vi "Word Wrap License File.vi"(8 "error in":errorcluster, 11 "txt file path":path) -> (0 "error out":errorcluster)   [LabVIEW 2011]
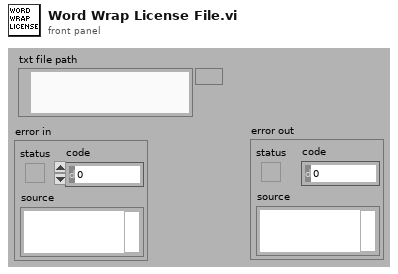
[diagram p1: front panel]
types:
  T1 = enum16{"User-specified Font", "Application Font", "System Font", "Dialog Font"}
  T2 = cluster{"Font Name:":string, "Size":i16, "Strikeout?":bool, "Italic?":bool, "Underline?":bool, "Outline?":bool, "Shadow?":bool, "Bold?":bool}
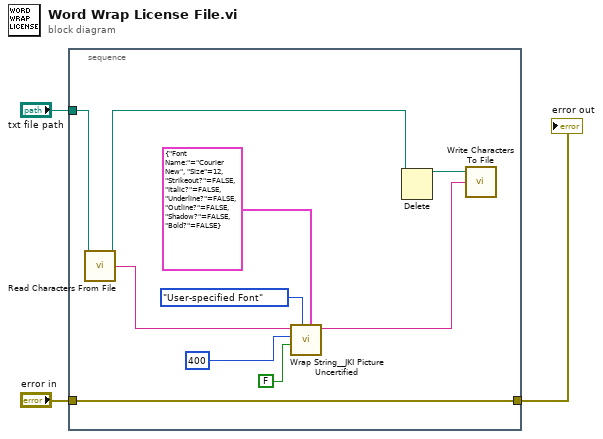
[diagram p0: block diagram]
diagram:
  n1 = stacked-sequence {
    tunnel: "txt file path" -> [w9]
    tunnel: [w4] -> w2
    tunnel: "error in" -> [w4]
    frame #0 {
      n2 = call <vilib>:"Read Characters From File.vi"("file path (dialog if empty)"=w9) -> ("new file path (NotAPath if cancelled)"=w7:path, "character string"=w8:string)  [unwired: 5 in, 2 out]
      n3 = call <vilib>:"Wrap String__JKI Picture Uncertified.vi"("[user-specified font]"=T2 {"Font Name:"="Courier New", "Size"=12, "Strikeout?"=FALSE, "Italic?"=FALSE, "Underline?"=FALSE, "Outline?"=FALSE, "Shadow?"=FALSE, "Bold?"=FALSE}, "desired font(Application)"=T1."User-specified Font", "Fast Algorithm? (T)"=FALSE, "Max Width"=400 ("Wrap length"), "String"=w8) -> ("Wrapped String"=w5:string)  [unwired: 5 in, 1 out]
      n4 = Delete(path (use dialog)=w7) -> (deleted path=w6:path)  [unwired: 4 in, 2 out]
      n5 = call <vilib>:"Write Characters To File.vi"("character string"=w5, "file path (dialog if empty)"=w6) -> ()  [unwired: 3 in, 1 out]
    }
  }
  "error out" <- w2
